vi "popUPConsultaListaRecetas.vi"(2 "listaRecetas":i32(listbox), 9 "ingresarLote":string="numLote", 10 "ingresarSteelGrade":string="numSteelGrade", 11 "ingresarOD":string="numeroOD") -> (3 "Listo ListarRecetas":bool=TRUE)   [LabVIEW 2014]
panel:
  in  "listarMejores10":bool
  in  "listarUltimas10":bool
  in  "textoFinCarga":string="Gracias por ingresar los datos del producto"
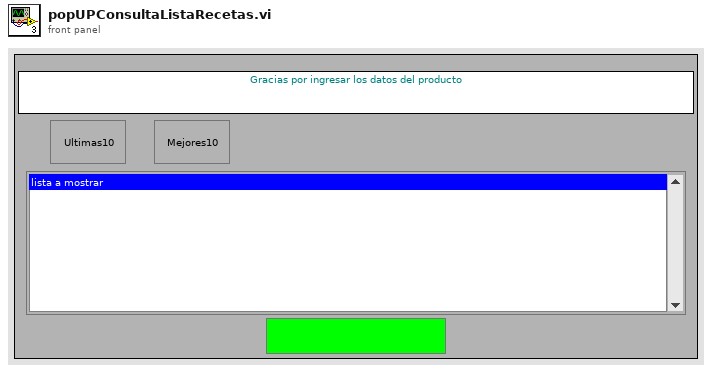
[diagram p1: front panel]
types:
  T1 = enum8{"Enabled", "Disabled", "Disabled and Grayed Out"}
  T2 = cluster{"queryAConsultar":string, "datosProducto":cluster{"OD":string, "SG":string, "LT":string}}
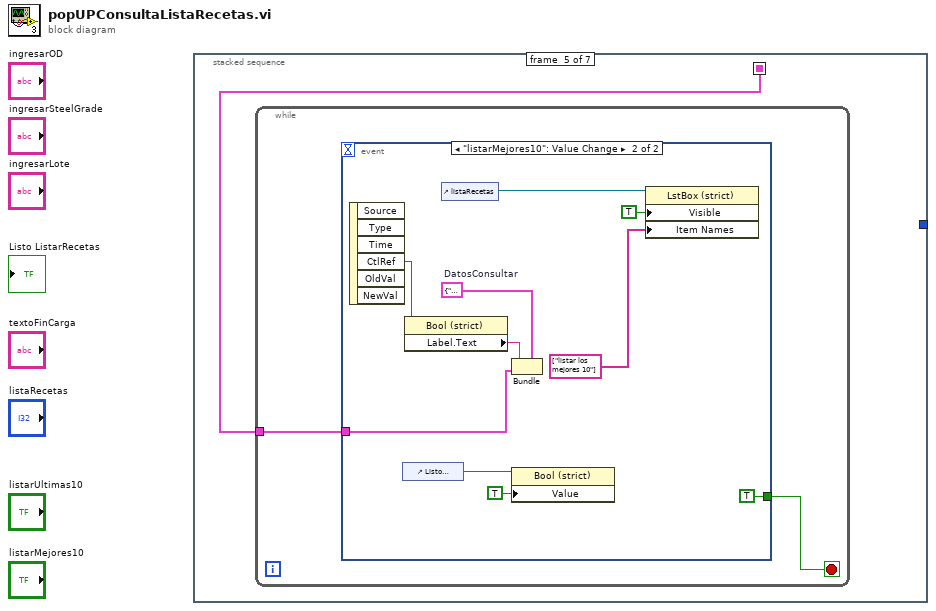
[diagram p0: block diagram]
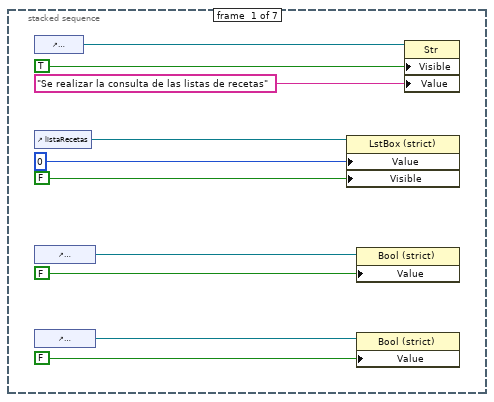
[diagram p2: hidden frame]
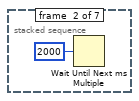
[diagram p3: hidden frame]
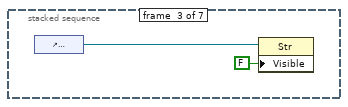
[diagram p4: hidden frame]
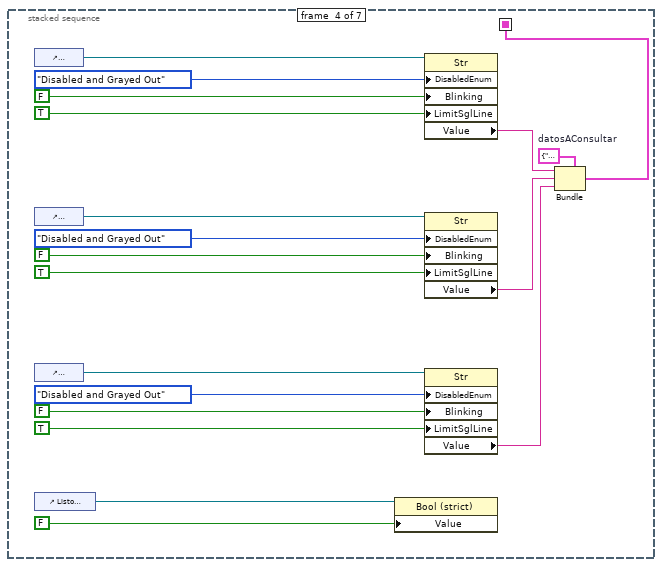
[diagram p5: hidden frame]
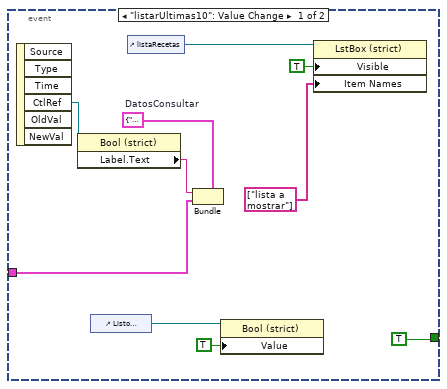
[diagram p6: hidden frame]
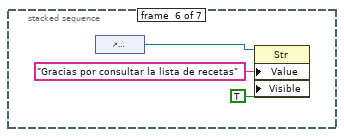
[diagram p7: hidden frame]
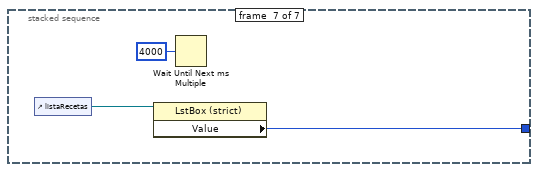
[diagram p8: hidden frame]
diagram:
  n1 = stacked-sequence {
    seq-local: [_ _ _ w14 _ _ _] -> [_ _ _ _ w33 _ _]
    tunnel: [_ _ _ _ _ _ w59] -> _
    frame #0 {
      n2 = control-ref of="textoFinCarga"() -> (w10:refnum<vi>)
      n3 = control-ref of="listaRecetas"() -> (w6:refnum<vi>)
      n4 = control-ref of="listarUltimas10"() -> (w4:refnum<vi>)
      n5 = control-ref of="listarMejores10"() -> (w2:refnum<vi>)
      n6 = property class="LstBox (strict)"(reference=w6, "Value"=0, "Visible"=FALSE) -> ()  [unwired: 1 in, 2 out]
      n7 = property class="Bool (strict)"(reference=w4, "Value"=FALSE) -> ()  [unwired: 1 in, 2 out]
      n8 = property class="Bool (strict)"(reference=w2, "Value"=FALSE) -> ()  [unwired: 1 in, 2 out]
      n9 = property class="Str"(reference=w10, "Visible"=TRUE, "Value"="Se realizar la consulta de las listas de recetas") -> ()  [unwired: 1 in, 2 out]
    }
    frame #1 {
      n10 = Wait Until Next ms Multiple(millisecond multiple=u32 2000) -> ()  [unwired: 1 out]
    }
    frame #2 {
      n11 = control-ref of="textoFinCarga"() -> (w13:refnum<vi>)
      n12 = property class="Str"(reference=w13, "Visible"=FALSE) -> ()  [unwired: 1 in, 2 out]
    }
    frame #3 {
      w15 = cluster{"OD":string, "SG":string, "LT":string} {"OD"="", "SG"="", "LT"=""}  # datosAConsultar
      n13 = control-ref of="ingresarOD"() -> (w32:refnum<vi>)
      n14 = control-ref of="ingresarSteelGrade"() -> (w30:refnum<vi>)
      n15 = control-ref of="ingresarLote"() -> (w28:refnum<vi>)
      n16 = control-ref of="Listo ListarRecetas"() -> (w21:refnum<vi>)
      n17 = property class="Bool (strict)"(reference=w21, "Value"=FALSE) -> ()  [unwired: 1 in, 2 out]
      n18 = property class="Str"(reference=w32, "DisabledEnum"=T1."Disabled and Grayed Out" ("Disabled"), "Blinking"=FALSE, "LimitSglLine"=TRUE ("Limit To Single Line?")) -> ("Value"=w18:string)  [unwired: 1 in, 2 out]
      n19 = property class="Str"(reference=w30, "DisabledEnum"=T1."Disabled and Grayed Out" ("Disabled"), "Blinking"=FALSE, "LimitSglLine"=TRUE ("Limit To Single Line?")) -> ("Value"=w17:string)  [unwired: 1 in, 2 out]
      n20 = property class="Str"(reference=w28, "DisabledEnum"=T1."Disabled and Grayed Out" ("Disabled"), "Blinking"=FALSE, "LimitSglLine"=TRUE ("Limit To Single Line?")) -> ("Value"=w16:string)  [unwired: 1 in, 2 out]
      n21 = Bundle(cluster=w15, "OD"=w18, "SG"=w17, "LT"=w16) -> (w14:cluster{"OD":string, "SG":string, "LT":string})
    }
    frame #4 {
      n22 = while {
        tunnel: w33 -> [w35]
        stop <- w34 stop-if-true
        n23 = event shown="[1] \"listarMejores10\": Value Change" {
          selector: _ -> [_ _]
          dyn-events: _ -> [_ _]
          timeout: _ -> [_ _]
          tunnel: w35 -> [w42 w52]
          tunnel: [TRUE TRUE] -> w34
          event "listarUltimas10": Value Change {
            w41 = T2 {"queryAConsultar"="", "datosProducto"={"OD"="", "SG"="", "LT"=""}}  # DatosConsultar
            n24 = event-data() -> ("CtlRef"=w44:refnum<vi>)  [unwired: 1 in, 5 out]
            n25 = property class="Bool (strict)"(reference=w44) -> ("Label.Text"=w43:string)  [unwired: 1 in, 2 out]
            n26 = control-ref of="Listo ListarRecetas"() -> (w37:refnum<vi>)
            n27 = control-ref of="listaRecetas"() -> (w40:refnum<vi>)
            n28 = Bundle(cluster=w41, "queryAConsultar"=w43, "datosProducto"=w42) -> ()  [unwired: 1 out]
            n29 = property class="Bool (strict)"(reference=w37, "Value"=TRUE) -> ()  [unwired: 1 in, 2 out]
            n30 = property class="LstBox (strict)"(reference=w40, "Visible"=TRUE, "Item Names"=string[] ["lista a mostrar"]) -> ()  [unwired: 1 in, 2 out]
          }
          event "listarMejores10": Value Change {
            w51 = T2 {"queryAConsultar"="", "datosProducto"={"OD"="", "SG"="", "LT"=""}}  # DatosConsultar
            n31 = event-data() -> ("CtlRef"=w54:refnum<vi>)  [unwired: 1 in, 5 out]
            n32 = control-ref of="Listo ListarRecetas"() -> (w47:refnum<vi>)
            n33 = property class="Bool (strict)"(reference=w54) -> ("Label.Text"=w53:string)  [unwired: 1 in, 2 out]
            n34 = control-ref of="listaRecetas"() -> (w50:refnum<vi>)
            n35 = Bundle(cluster=w51, "queryAConsultar"=w53, "datosProducto"=w52) -> ()  [unwired: 1 out]
            n36 = property class="Bool (strict)"(reference=w47, "Value"=TRUE) -> ()  [unwired: 1 in, 2 out]
            n37 = property class="LstBox (strict)"(reference=w50, "Visible"=TRUE, "Item Names"=string[] ["listar los mejores 10"]) -> ()  [unwired: 1 in, 2 out]
          }
        }
      }
    }
    frame #5 {
      n38 = control-ref of="textoFinCarga"() -> (w58:refnum<vi>)
      n39 = property class="Str"(reference=w58, "Value"="Gracias por consultar la lista de recetas", "Visible"=TRUE) -> ()  [unwired: 1 in, 2 out]
    }
    frame #6 {
      n40 = control-ref of="listaRecetas"() -> (w60:refnum<vi>)
      n41 = property class="LstBox (strict)"(reference=w60) -> ("Value"=w59:i32)  [unwired: 1 in, 2 out]
      n42 = Wait Until Next ms Multiple(millisecond multiple=u32 4000) -> ()  [unwired: 1 out]
    }
  }
